vi "MatrixB_Vg_dep_Tdep.vi"(0 "T-table String":string, 3 "Time Stamp":timestamp, 6 "Play Button":bool, 7 "Custom Folder":string, 8 "Settings":T3={"Ring 3"=1, "Ring 2"=4, "Fixed Current mkA"=0.5, "If yes, the current is:"=enum."Radio Selection 1", "Ressitance measurements?"=TRUE, "Commute DC current?"=FALSE} {"Ring 3" items=["1 kOhm", "10 kOhm", "100 kOhm", "1 Mohm", "10 mOhm"]; "Ring 2" items=["1 kOhm", "10 kOhm", "100 kOhm", "1 Mohm", "10 MOhm"]}, 9 "Instruments":T4={"Oscillator"=TRUE, "Addr 1 lock-in"=TRUE, "Addr 1 lock-in oop"=TRUE, "Addr 2 lock-in"=TRUE, "Addr 2 lock-in oop"=TRUE, "Addr 3 lock-in"=FALSE, "Addr 3 lock-in oop"=FALSE, "Voltage (Vk1)"=FALSE, "Current (Ik1)"=TRUE, "Voltage (Vk2)"=FALSE, "Current (Ik2)"=FALSE, "Voltage (Vk3)"=FALSE, "Current (Ik3)"=FALSE, "Channel 1 (Vnano1)  "=FALSE, "Channel 2 (Vnano1b)"=FALSE, "Channel 1 (Vnano2)   "=FALSE, "Channel 2 (Vnano2b)"=FALSE, "Thermometer 1 (T1)"=TRUE, "Magnetic Field (B)"=TRUE, "Capacitance (C) and Loss (L)"=FALSE}, 10 "BCluster":T5={"B1 (V)"=-1.0, "B2 (V)"=1.0, "Sweep rate, T/min"=0.3, "Time btw \npoints, sec"=1.0, "No-record rate, T/min"=0.5, "Full sweep?"=FALSE, "Odd confgurations"=TRUE} {"No-record rate, T/min" min=0.0 max=1.0 step=0.01 format="%_4f"; "B2 (V)" min=-4.0 max=4.0 step=0.1 format="%.2f"; "Time btw \npoints, sec" format="%.2f"; "Sweep rate, T/min" min=0.0 max=1.0 step=0.01 format="%_4f"; "B1 (V)" min=-4.0 max=4.0 step=0.1 format="%.2f"}, 11 "TCluster":T2={"Starting T (K)"=30.0, "Final T (K)"=100.0, "Step (T)"=1.0, "Stabilisation , min"=1.0, "Wait 1st point?"=FALSE, "At the end:"=TRUE} {"Final T (K)" min=-4.0 max=4.0 step=0.1 format="%.2f"; "Stabilisation , min" format="%.2f"; "Step (T)" min=0.0 max=1.0 step=0.01 format="%_4f"; "Starting T (K)" min=-4.0 max=4.0 step=0.1 format="%.2f"}) -> ()   [LabVIEW 2017]
uses:
  <vilib>/Utility/file.llb/Read From Spreadsheet File (DBL).vi
panel:
  in  "Vg-table String":string
  out "Vg Array":dbl[](array[numeric])
  in  "VgCluster":T1={"Starting Vg (V)"=-1.0, "Final Vg (V)"=1.0, "Step (V)"=1.0} {"Final Vg (V)" min=-4.0 max=4.0 step=0.1 format="%.2f"; "Step (V)" min=0.0 max=1.0 step=0.01 format="%_4f"; "Starting Vg (V)" min=-4.0 max=4.0 step=0.1 format="%.2f"}
  in  "No record Vg rate (V/min)":dbl=150.0
  out "Communication":string
  out "T Array":dbl[](array[numeric])
  out "Experiment ends at:":string
  out "Hours":dbl format="%.1f"
  out "Estimated time of experiment:":i16
  out "ArraySens":i8[](array[numeric])
  out "ArrayOsc":dbl[](array[numeric])
  out "# of configurations":i8
  out "Large Array":bool[][][](array[boolean])
  out "Contact configuration file (*.conf)":path
  # "1"
  # "hours"
  # "min.="
  # "Values of T can be also entered as the \ntable by copying and pasting a column \nof numbers in a \"T table\" string at the \nfar right side of this window."
  # "Lock-in Amplifiers"
  # "Temperature"
  # "SourceMeters"
  # "Nanovoltmeters"
  # "Main"
  # "(not recommended, too slow)"
  # "Magnetic Field"
  # "Capacitance & Loss"
  # "(not recommended, too slow)"
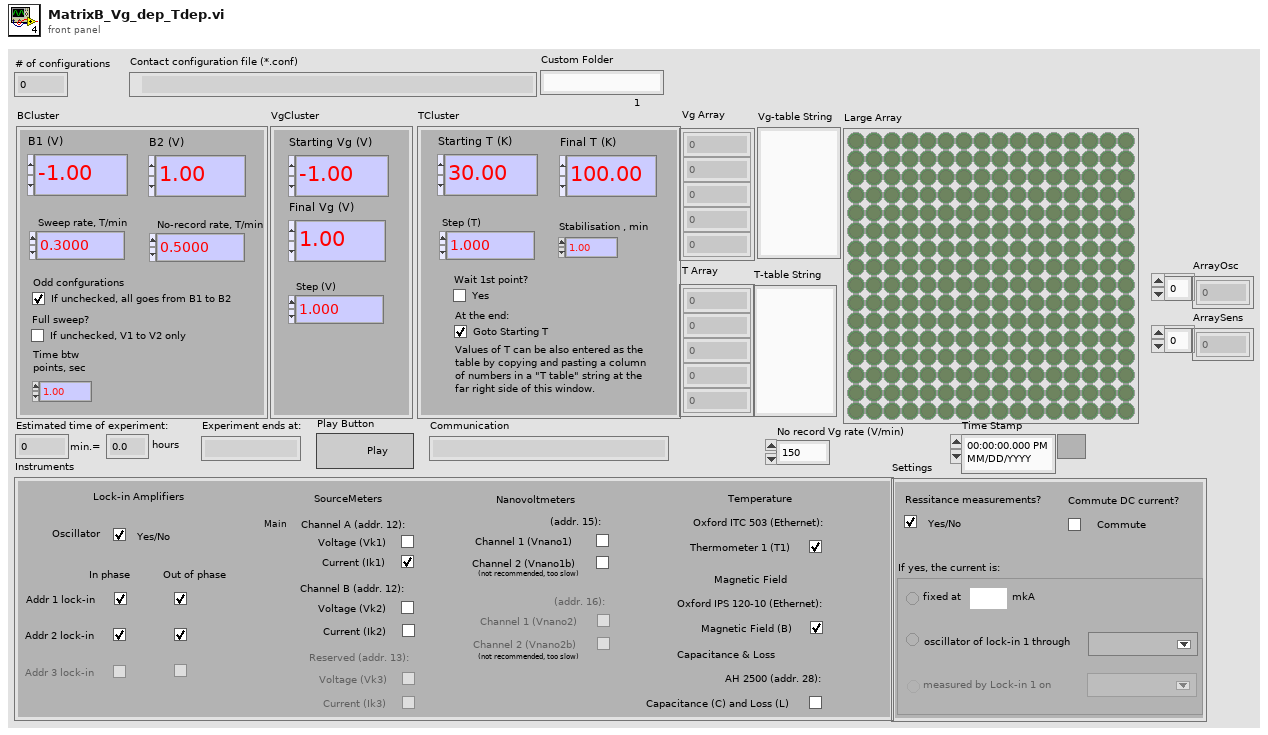
[diagram p1: front panel]
types:
  T1 = cluster{"Starting Vg (V)":dbl, "Final Vg (V)":dbl, "Step (V)":dbl}
  T2 = cluster{"Starting T (K)":dbl, "Final T (K)":dbl, "Step (T)":dbl, "Stabilisation , min":dbl, "Wait 1st point?":bool, "At the end:":bool}
  T3 = cluster{"Ring 3":u16, "Ring 2":u16, "Fixed Current mkA":dbl, "If yes, the current is:":enum32{"Radio Selection 1", "Radio Selection 2", "Radio Selection 3"}, "Ressitance measurements?":bool, "Commute DC current?":bool}
  T4 = cluster{"Oscillator":bool, "Addr 1 lock-in":bool, "Addr 1 lock-in oop":bool, "Addr 2 lock-in":bool, "Addr 2 lock-in oop":bool, "Addr 3 lock-in":bool, "Addr 3 lock-in oop":bool, "Voltage (Vk1)":bool, "Current (Ik1)":bool, "Voltage (Vk2)":bool, "Current (Ik2)":bool, "Voltage (Vk3)":bool, "Current (Ik3)":bool, "Channel 1 (Vnano1)  ":bool, "Channel 2 (Vnano1b)":bool, "Channel 1 (Vnano2)   ":bool, "Channel 2 (Vnano2b)":bool, "Thermometer 1 (T1)":bool, "Magnetic Field (B)":bool, "Capacitance (C) and Loss (L)":bool}
  T5 = cluster{"B1 (V)":dbl, "B2 (V)":dbl, "Sweep rate, T/min":dbl, "Time btw \npoints, sec":dbl, "No-record rate, T/min":dbl, "Full sweep?":bool, "Odd confgurations":bool}
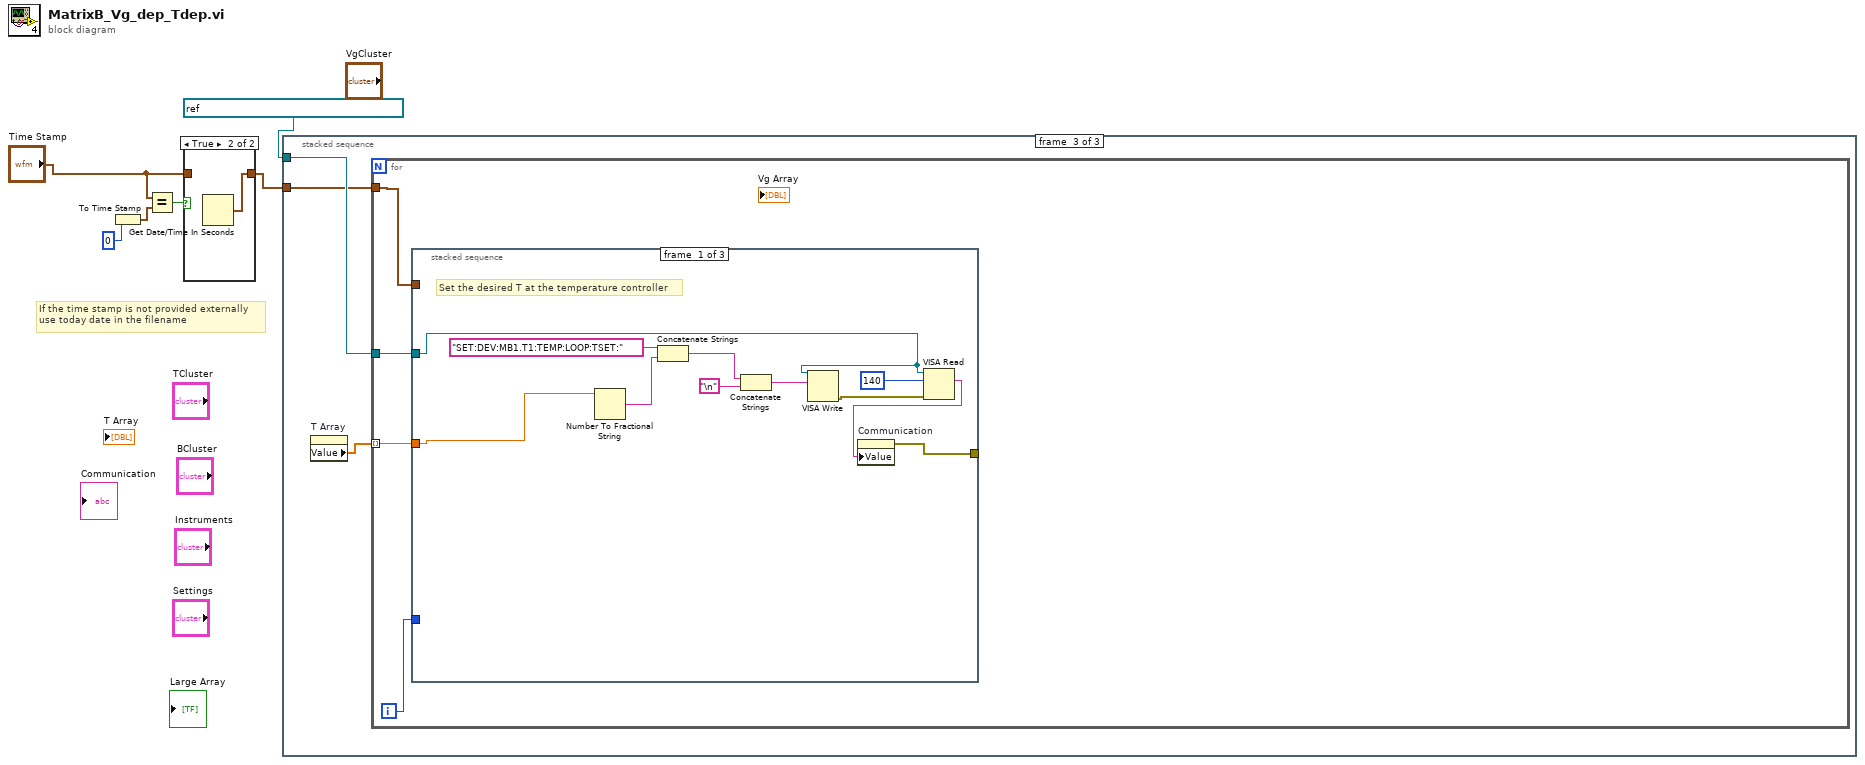
[diagram p0: block diagram]
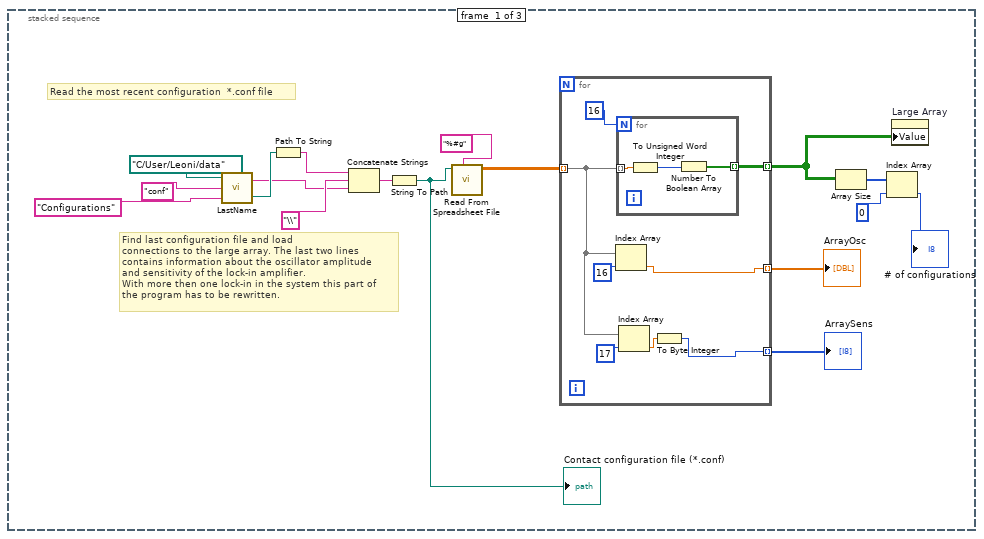
[diagram p3: hidden frame]
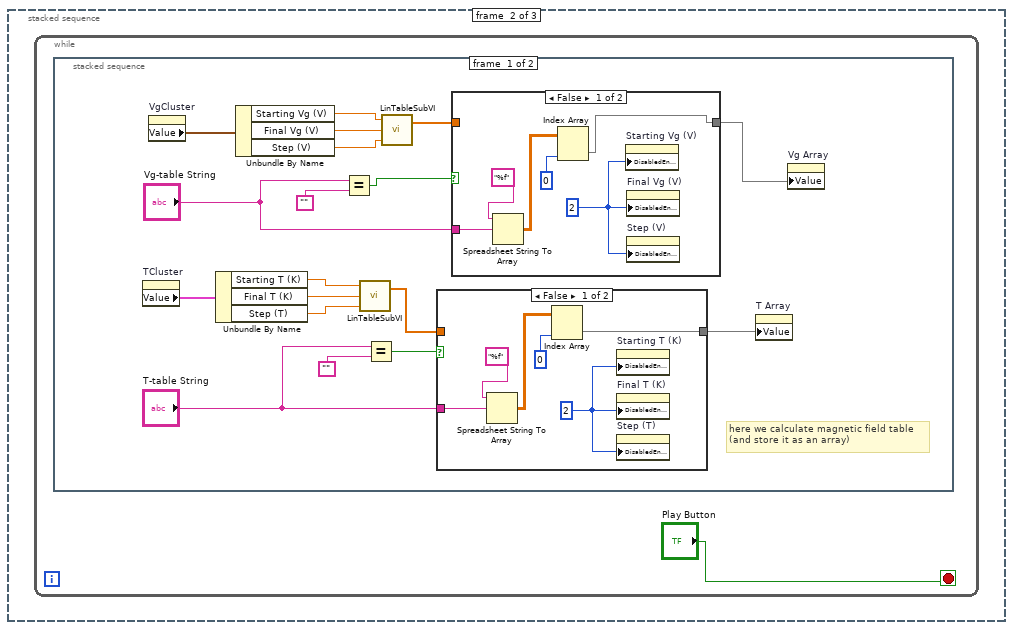
[diagram p4: hidden frame]
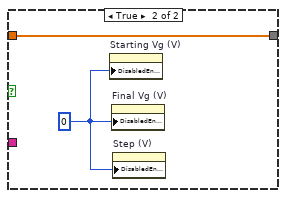
[diagram p5: hidden frame]
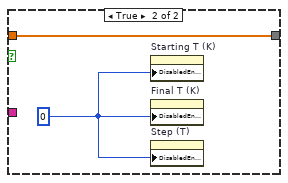
[diagram p6: hidden frame]
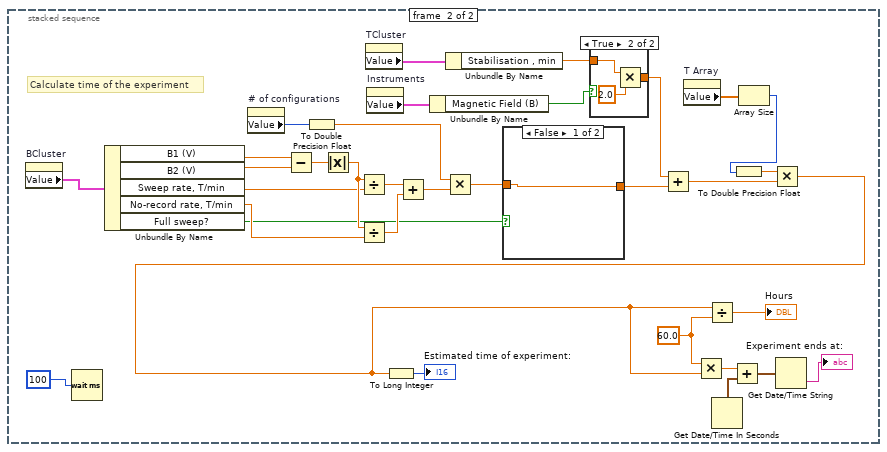
[diagram p7: hidden frame]
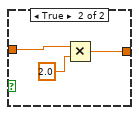
[diagram p9: hidden frame]
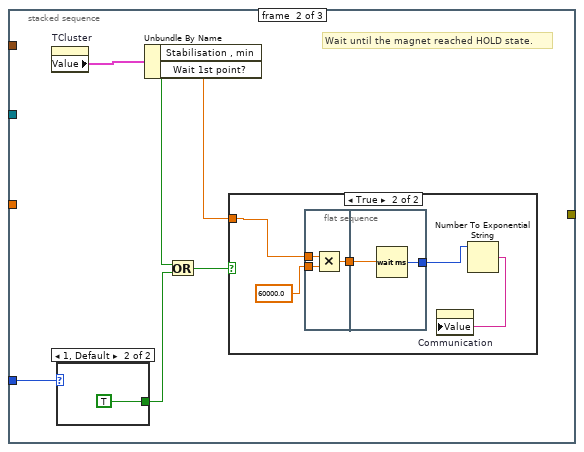
[diagram p10: hidden frame]
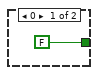
[diagram p12: hidden frame]
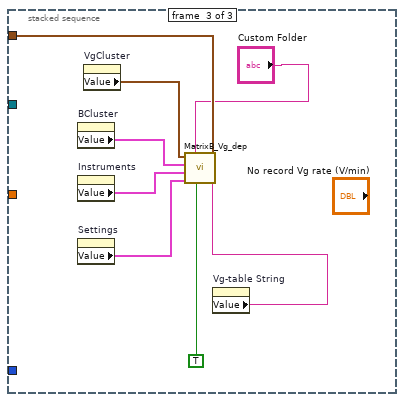
[diagram p13: hidden frame]
diagram:
  # "If the time stamp is not provided externally\nuse today date in the filename"
  n1 = To Time Stamp(1:0) -> (0:w5:timestamp)
  n2 = Equal?(x="Time Stamp", y=w5) -> (x = y?=w4:bool)
  n3 = case shown="True" w4 {
    tunnel: "Time Stamp" -> [w7 _]
    tunnel: [w7 w8] -> w2
    frame False {
    }
    frame True {
      n4 = Get Date/Time In Seconds() -> (seconds since 1Jan1904=w8:timestamp)
    }
  }
  n5 = stacked-sequence {
    tunnel: w2 -> [_ _ w113]
    tunnel: refnum<visa-resource-name> "TCPIP0::192.168.128.2::7020::SOCKET" ("VISA resource name") -> [_ _ w115]
    frame #0 {
      # "Read the most recent configuration  *.conf file"
      # "Find last configuration file and load \nconnections to the large array. The last two lines \ncontains information about the oscillator amplitude\nand sensitivity of the lock-in amplifier.\nWith more then one lock-in in the system this part of \nthe program has to be rewritten."
      n6 = call "LastName.vi"("Custom Folder"="Configurations", "Extention"="conf", "User Data Folder"=path "C:/User/Leoni/data") -> ("created path"=w21:path, "String"=w20:string)
      n7 = Path To String(path=w21) -> (string=w25:string)
      n8 = Concatenate Strings(w25, "\\", w20) -> (w23:string)
      n9 = String To Path(string=w23) -> (path=w11:path)
      "Contact configuration file (*.conf)" <- w11
      n10 = call-poly <vilib>:"Read From Spreadsheet File.vi"("format (%.3f)"="%#g", "file path (dialog if empty)"=w11) -> ("all rows"=w16:dbl[][])  [unwired: 5 in, 4 out]
      n11 = for {
        tunnel: w16 -> [w29] mode=indexing
        tunnel: [w33] -> w13 mode=indexing
        tunnel: [w28] -> w10 mode=indexing
        tunnel: [w27] -> w9 mode=indexing
        n12 = Index Array(array=w29, index=16) -> (element=w28:dbl)
        n13 = for {
          N: 16 -> [_]
          tunnel: w29 -> [w36] mode=indexing
          tunnel: [w34] -> w33 mode=indexing
          n14 = To Unsigned Word Integer(number=w36) -> (unsigned 16bit integer=w35:u16)
          n15 = Number To Boolean Array(number=w35) -> (Boolean array=w34:bool[])
        }
        n16 = Index Array(array=w29, index=17) -> (element=w30:dbl)
        n17 = To Byte Integer(number=w30) -> (8bit integer=w27:i8)
      }
      "ArrayOsc" <- w10
      "ArraySens" <- w9
      n18 = Array Size(array=w13) -> (size(s)=w15:i32[])
      n19 = Index Array(array=w15, index=0) -> (element=→"# of configurations":i32)
      n20 = property on="Large Array" class="Arr (strict)"("Value"=w13) -> ()  [unwired: 2 in, 2 out]
    }
    frame #1 {
      n21 = while {
        stop <- "Play Button" stop-if-true
        n22 = stacked-sequence {
          frame #0 {
            # "here we calculate magnetic field table\n(and store it as an array)"
            n23 = property on="TCluster" class="Clust (strict)"() -> ("Value"=w51:T2)  [unwired: 2 in, 2 out]
            n24 = property on="VgCluster" class="Clust (strict)"() -> ("Value"=w46:T1)  [unwired: 2 in, 2 out]
            n25 = Unbundle By Name(w51) -> ("Starting T (K)"=w50:dbl, "Final T (K)"=w49:dbl, "Step (T)"=w48:dbl)
            n26 = Unbundle By Name(w46) -> ("Starting Vg (V)"=w45:dbl, "Final Vg (V)"=w44:dbl, "Step (V)"=w43:dbl)
            n27 = Equal?(x="Vg-table String", y="") -> (x = y?=w41:bool)
            n28 = call "LinTableSubVI.vi"("Step"=w48, "Final"=w49, "Initial"=w50) -> ("Array"=w55:dbl[])  [unwired: 1 in]
            n29 = Equal?(x="T-table String", y="") -> (x = y?=w52:bool)
            n30 = call "LinTableSubVI.vi"("Step"=w43, "Final"=w44, "Initial"=w45) -> ("Array"=w40:dbl[])  [unwired: 1 in]
            n31 = case shown="False" w52 {
              tunnel: [w66 w71] -> w47
              tunnel: w55 -> [_ w71]
              tunnel: "T-table String" -> [w65 _]
              frame False {
                w64 = 2
                n32 = Spreadsheet String To Array(format string="%f", spreadsheet string=w65) -> (array=w68:dbl[][])  [unwired: 2 in]
                n33 = Index Array(array=w68, index (col)=0) -> (element=w66:dbl[])  [unwired: 1 in]
                n34 = property on="Starting T (K)" class="DigNum (strict)"("DisabledEnum"=w64) -> ()  [unwired: 2 in, 2 out]
                n35 = property on="Final T (K)" class="DigNum (strict)"("DisabledEnum"=w64) -> ()  [unwired: 2 in, 2 out]
                n36 = property on="Step (T)" class="DigNum (strict)"("DisabledEnum"=w64) -> ()  [unwired: 2 in, 2 out]
              }
              frame True {
                w70 = 0
                n37 = property on="Starting T (K)" class="DigNum (strict)"("DisabledEnum"=w70) -> ()  [unwired: 2 in, 2 out]
                n38 = property on="Final T (K)" class="DigNum (strict)"("DisabledEnum"=w70) -> ()  [unwired: 2 in, 2 out]
                n39 = property on="Step (T)" class="DigNum (strict)"("DisabledEnum"=w70) -> ()  [unwired: 2 in, 2 out]
              }
            }
            n40 = case shown="False" w41 {
              tunnel: [w56 w62] -> w38
              tunnel: w40 -> [_ w62]
              tunnel: "Vg-table String" -> [w58 _]
              frame False {
                w57 = 2
                n41 = Spreadsheet String To Array(format string="%f", spreadsheet string=w58) -> (array=w60:dbl[][])  [unwired: 2 in]
                n42 = Index Array(array=w60, index (col)=0) -> (element=w56:dbl[])  [unwired: 1 in]
                n43 = property on="Starting Vg (V)" class="DigNum (strict)"("DisabledEnum"=w57) -> ()  [unwired: 2 in, 2 out]
                n44 = property on="Final Vg (V)" class="DigNum (strict)"("DisabledEnum"=w57) -> ()  [unwired: 2 in, 2 out]
                n45 = property on="Step (V)" class="DigNum (strict)"("DisabledEnum"=w57) -> ()  [unwired: 2 in, 2 out]
              }
              frame True {
                w63 = 0
                n46 = property on="Starting Vg (V)" class="DigNum (strict)"("DisabledEnum"=w63) -> ()  [unwired: 2 in, 2 out]
                n47 = property on="Final Vg (V)" class="DigNum (strict)"("DisabledEnum"=w63) -> ()  [unwired: 2 in, 2 out]
                n48 = property on="Step (V)" class="DigNum (strict)"("DisabledEnum"=w63) -> ()  [unwired: 2 in, 2 out]
              }
            }
            n49 = property on="T Array" class="Arr (strict)"("Value"=w47) -> ()  [unwired: 2 in, 2 out]
            n50 = property on="Vg Array" class="Arr (strict)"("Value"=w38) -> ()  [unwired: 2 in, 2 out]
          }
          frame #1 {
            w84 = 60.0
            # "Calculate time of the experiment"
            n51 = property on="BCluster" class="Clust (strict)"() -> ("Value"=w103:T5)  [unwired: 2 in, 2 out]
            n52 = Wait (ms)(milliseconds to wait=100) -> ()  [unwired: 1 out]
            n53 = Unbundle By Name(w103) -> ("B1 (V)"=w102:dbl, "B2 (V)"=w101:dbl, "Sweep rate, T/min"=w98:dbl, "No-record rate, T/min"=w97:dbl, "Full sweep?"=w91:bool)
            n54 = property on="# of configurations" class="DigNum (strict)"() -> ("Value"=w93:i8)  [unwired: 2 in, 2 out]
            n55 = Subtract(x=w102, y=w101) -> (x-y=w100:dbl)
            n56 = To Double Precision Float(number=w93) -> (double precision float=w92:dbl)
            n57 = Absolute Value(x=w100) -> (abs(x)=w99:dbl)
            n58 = Divide(x=w99, y=w98) -> (x/y=w96:dbl)
            n59 = Divide(x=w99, y=w97) -> (x/y=w95:dbl)
            n60 = property on="TCluster" class="Clust (strict)"() -> ("Value"=w80:T2)  [unwired: 2 in, 2 out]
            n61 = property on="Instruments" class="Clust (strict)"() -> ("Value"=w75:T4)  [unwired: 2 in, 2 out]
            n62 = Add(x=w96, y=w95) -> (x+y=w94:dbl)
            n63 = Unbundle By Name(w75) -> ("Magnetic Field (B)"=w74:bool)
            n64 = Multiply(x=w92, y=w94) -> (x*y=w90:dbl)
            n65 = Unbundle By Name(w80) -> ("Stabilisation , min"=w73:dbl)
            n66 = case shown="False" w91 {
              tunnel: w90 -> [w109 w112]
              tunnel: [w109 w110] -> w81
              frame False {
              }
              frame True {
                n67 = Multiply(x=w112, y=2.0) -> (x*y=w110:dbl)
              }
            }
            n68 = case shown="True" w74 {
              tunnel: w73 -> [w105 w107]
              tunnel: [w105 w106] -> w72
              frame False {
              }
              frame True {
                n69 = Multiply(x=w107, y=2.0) -> (x*y=w106:dbl)
              }
            }
            n70 = Add(x=w72, y=w81) -> (x+y=w79:dbl)
            n71 = property on="T Array" class="Arr (strict)"() -> ("Value"=w82:dbl[])  [unwired: 2 in, 2 out]
            n72 = Get Date/Time In Seconds() -> (seconds since 1Jan1904=w88:timestamp)
            n73 = Array Size(array=w82) -> (size(s)=w77:i32)
            n74 = To Double Precision Float(number=w77) -> (double precision float=w78:dbl)
            n75 = Multiply(x=w78, y=w79) -> (x*y=w76:dbl)
            n76 = To Long Integer(number=w76) -> (32bit integer=→"Estimated time of experiment:":i32)
            n77 = Multiply(x=w84, y=w76) -> (x*y=w83:dbl)
            n78 = Divide(x=w76, y=w84) -> (x/y=→"Hours":dbl)
            n79 = Add(x=w83, y=w88) -> (x+y=w87:timestamp)
            n80 = Get Date/Time String(seconds (now)=w87) -> (time string=→"Experiment ends at:":string)  [unwired: 2 in, 1 out]
          }
        }
      }
    }
    frame #2 {
      n81 = property on="T Array" class="Arr (strict)"() -> ("Value"=w114:dbl[])  [unwired: 2 in, 2 out]
      n82 = for {
        tunnel: w115 -> [w119]
        tunnel: w114 -> [w118] mode=indexing
        tunnel: w113 -> [w116]
        i -> [w117]
        n83 = stacked-sequence {
          tunnel: w119 -> [w122 _ _]
          tunnel: w118 -> [w120 _ _]
          tunnel: [w130 _ _] -> _
          tunnel: w117 -> [_ w134 _]
          tunnel: w116 -> [_ _ w152]
          frame #0 {
            # "Set the desired T at the temperature controller"
            n84 = Number To Fractional String(number=w120) -> (F-format string=w128:string)  [unwired: 3 in]
            n85 = Concatenate Strings("SET:DEV:MB1.T1:TEMP:LOOP:TSET:" ("string"), w128) -> (w123:string)
            n86 = Concatenate Strings(w123, "\n") -> (w124:string)
            n87 = VISA Write(VISA resource name=w122, write buffer=w124) -> (error out=w127:errorcluster)  [unwired: 1 in, 2 out]
            n88 = VISA Read(VISA resource name=w122, byte count=140, error in (no error)=w127) -> (read buffer=w121:string)  [unwired: 3 out]
            n89 = property on="Communication" class="Str"("Value"=w121) -> (error out=w130:errorcluster)  [unwired: 2 in, 1 out]
          }
          frame #1 {
            # "Wait until the magnet reached HOLD state."
            n90 = property on="TCluster" class="Clust (strict)"() -> ("Value"=w136:T2)  [unwired: 2 in, 2 out]
            n91 = case shown="1, Default" w134 {
              tunnel: [FALSE TRUE] -> w132
              frame 0 {
              }
              frame 1, Default {
              }
            }
            n92 = Unbundle By Name(w136) -> ("Stabilisation , min"=w135:dbl, "Wait 1st point?"=w133:bool)
            n93 = Or(x=w133, y=w132) -> (x .or. y?=w131:bool)
            n94 = case shown="True" w131 {
              tunnel: w135 -> [_ w139]
              frame False {
              }
              frame True {
                n95 = flat-sequence {
                  tunnel: w139 -> [w144]
                  tunnel: 60000.0 -> [w143]
                  tunnel: [w142] -> w137
                  tunnel: [w146] -> w140
                  tunnel: w137 -> [w145]
                  frame #0 {
                    n96 = Multiply(x=w144, y=w143) -> (x*y=w142:dbl)
                  }
                  frame #1 {
                    n97 = Wait (ms)(milliseconds to wait=w145) -> (millisecond timer value=w146:u32)
                  }
                }
                n98 = Number To Exponential String(number=w140) -> (E-format string=w141:string)  [unwired: 3 in]
                n99 = property on="Communication" class="Str"("Value"=w141) -> ()  [unwired: 2 in, 2 out]
              }
            }
          }
          frame #2 {
            n100 = property on="BCluster" class="Clust (strict)"() -> ("Value"=w156:T5)  [unwired: 2 in, 2 out]
            n101 = property on="Instruments" class="Clust (strict)"() -> ("Value"=w153:T4)  [unwired: 2 in, 2 out]
            n102 = property on="Settings" class="Clust (strict)"() -> ("Value"=w154:T3)  [unwired: 2 in, 2 out]
            n103 = property on="VgCluster" class="Clust (strict)"() -> ("Value"=w151:T1)  [unwired: 2 in, 2 out]
            n104 = property on="Vg-table String" class="Str"() -> ("Value"=w149:string)  [unwired: 2 in, 2 out]
            n105 = call "MatrixB_Vg_dep.vi"("Vg-table String"=w149, "Time Stamp"=w152, "Play Button"=TRUE, "Custom Folder"="Custom Folder", "Settings"=w154, "Instruments"=w153, "BCluster"=w156, "VgCluster"=w151) -> ()  [unwired: 4 in]
          }
        }
      }
    }
  }
